vi "SLL DE Cross Check AO Channels with Type Def.vi"(8 "error in (no error)":errorcluster, 10 "AO Channel Name (Type def)":string[](array[string]), 11 "AO Virtial Channels Info":string[](array[string])) -> (0 "error out":errorcluster)   [LabVIEW 2013]
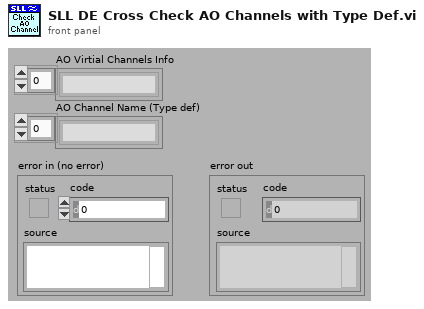
[diagram p1: front panel]
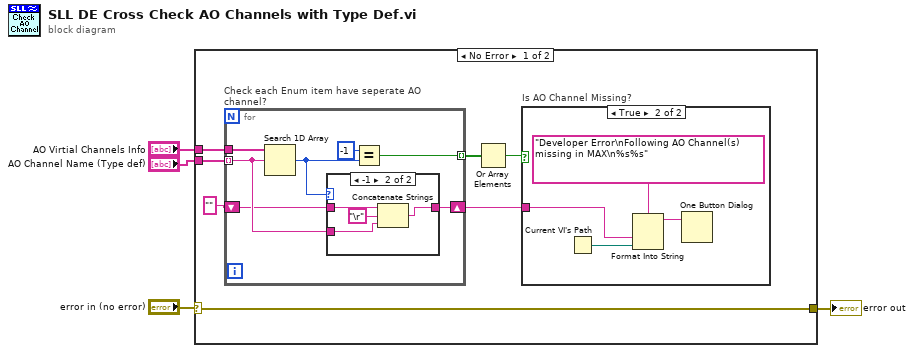
[diagram p0: block diagram]
diagram:
  n1 = case shown="No Error" "error in (no error)" {
    selector: "error in (no error)" -> [w5 w28]
    tunnel: "AO Virtial Channels Info" -> [w7 _]
    tunnel: "AO Channel Name (Type def)" -> [w6 _]
    tunnel: [w5 w28] -> w1
    frame No Error {
      n2 = for "Check each Enum item have seperate AO channel?" {
        tunnel: w6 -> [w20] mode=indexing
        tunnel: w7 -> [w22]
        tunnel: [w21] -> w11 mode=indexing
        shift-right: [w19] -> w8
        shift-left: "" -> [w18]
        n3 = Search 1D Array(1D array=w22, element=w20) -> (index of element=w17:i32)  [unwired: 1 in]
        n4 = case shown="-1" w17 {
          tunnel: w20 -> [_ w26]
          tunnel: [w23 w25] -> w19
          tunnel: w18 -> [w23 w24]
          frame Default {
          }
          frame -1 {
            n5 = Concatenate Strings(w24, "\r", w26) -> (w25:string)
          }
        }
        n6 = Equal?(x=-1 ("y"), y=w17) -> (x = y?=w21:bool)
      }
      n7 = Or Array Elements(Boolean array=w11) -> (logical OR=w10:bool)
      n8 = case "Is AO Channel Missing?" shown="True" w10 {
        tunnel: w8 -> [_ w12]
        frame False {
        }
        frame True {
          n9 = Current VI's Path() -> (path=w13:path)
          n10 = Format Into String(format string="Developer Error\nFollowing AO Channel(s) missing in MAX\n%s%s" ("message"), w12, w13) -> (resulting string=w14:string)  [unwired: 2 in, 1 out]
          n11 = One Button Dialog(message=w14) -> ()  [unwired: 1 in, 1 out]
        }
      }
    }
    frame Error {
    }
  }
  "error out" <- w1
